vi "02 A_Setting a servo.vi"() -> ()   [LabVIEW 2019]
uses:
  _Subs/OpenDiagram/Open_XControl.xctl
  <vilib>/Instr/_visa.llb/VISA Configure Serial Port (Instr).vi
panel:
  in  "OpenDiag":refnum<vi>(xcontrol)
  out "position read":u8=100
  in  "Position":u8(slide)=98 scale=0.0..180.0
  in  "Arduino code":string="// include the Servo library\n#include <Servo.h>\n\nServo myServo;  // create a servo object\n\nvoid setup() {\n  myServo.attach(9); // attaches the servo on pin 9 to the servo object\n  Serial.begin(9600);\n\n}\n\nvoid loop() {   \n  int incomingByte;\n  if (Serial.available() > 0) {\n    int incomingByte = Serial.read();\n    myServo.write(incomingByte);\n    Serial.write(incomingByte);\n  }\n}"
  in  "stop":bool
  out "Connected":bool
  in  "Arduino Port":refnum<visa-resource-name>="ASRL26::INSTR"
  # "02 Arduino Setting  a Servo\nThis code takes will send a setting to your Arduino\n\nInstructions:\n1. Download the Arduino Code (SimpelServo) into your Arduino using the Arduino IDE\n2. Select the Arduino port \n3. Hit Run - and move the position slider"
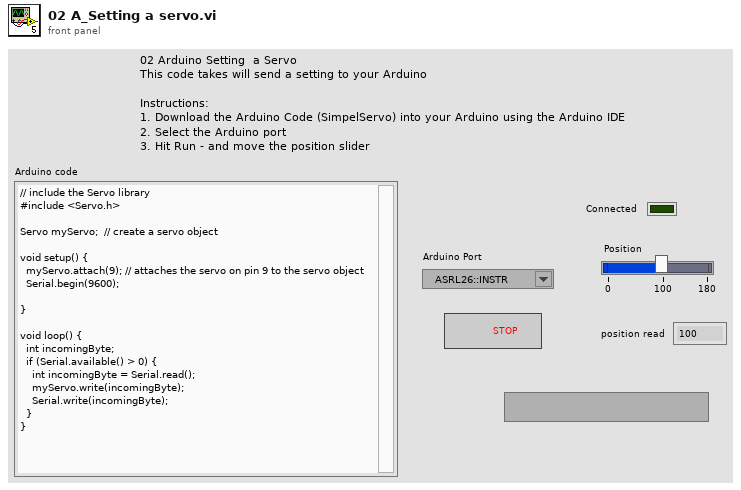
[diagram p1: front panel]
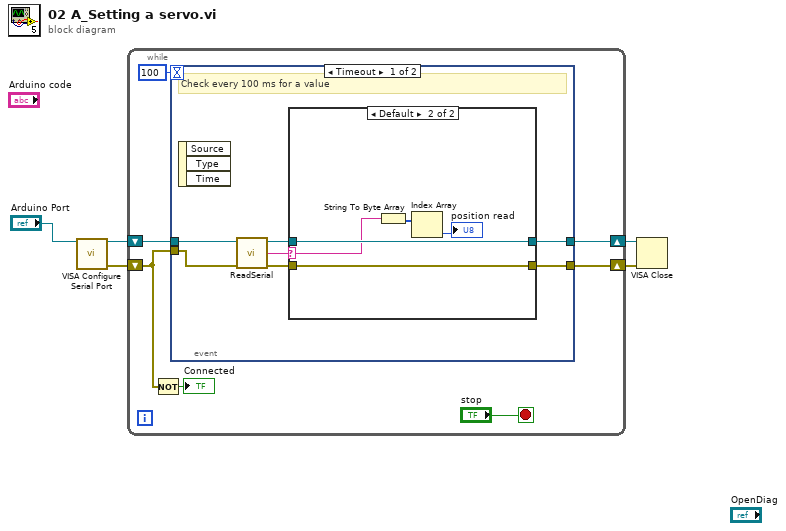
[diagram p0: block diagram]
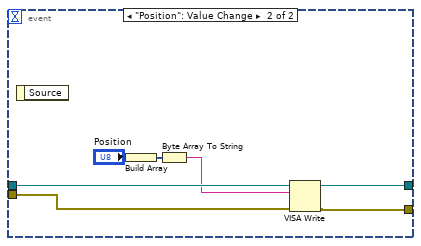
[diagram p3: hidden frame]
diagram:
  n1 = call-poly "VISA Configure Serial Port"("VISA resource name"="Arduino Port") -> ("VISA resource name out"=w4:refnum<visa-resource-name>, "error out"=w3:errorcluster)  [unwired: 13 in]
  n2 = while {
    shift-right: [w10] -> w1
    shift-left: w4 -> [w12]
    shift-right: [w11] -> w2
    shift-left: w3 -> [w8]
    stop <- "stop" stop-if-true
    n3 = Not(x=w8) -> (.not. x?=→"Connected":bool)
    n4 = event shown="[0] Timeout" {
      selector: _ -> [_ _]
      dyn-events: _ -> [_ _]
      timeout: 100 -> [_ _]
      tunnel: w12 -> [w17 w33]
      tunnel: [w19 w31] -> w11
      tunnel: [w18 w30] -> w10
      tunnel: w8 -> [w16 w32]
      event Timeout {
        # "Check every 100 ms for a value"
        n5 = event-data() -> ()  [unwired: 1 in, 3 out]
        n6 = call "ReadSerial.vi"("error in (no error)"=w16, "VISA Refnum in"=w17) -> ("error out"=w14:errorcluster, "String"=w13:string, "VISA Refnum out"=w15:refnum<visa-resource-name>)  [unwired: 7 in]
        n7 = case shown="Default" w13 {
          selector: w13 -> [_ w22]
          tunnel: [w20 w23] -> w19
          tunnel: [w21 w24] -> w18
          tunnel: w15 -> [w21 w24]
          tunnel: w14 -> [w20 w23]
          frame "" {
          }
          frame Default {
            n8 = String To Byte Array(string=w22) -> (unsigned byte array=w26:u8[])
            n9 = Index Array(array=w26) -> (element=→"position read":u8)  [unwired: 1 in]
          }
        }
      }
      event "Position": Value Change {
        n10 = event-data() -> ()  [unwired: 1 in, 1 out]
        n11 = Build Array("Position") -> (w28:u8[])
        n12 = Byte Array To String(unsigned byte array=w28) -> (string=w27:string)
        n13 = VISA Write(VISA resource name=w33, write buffer=w27, error in (no error)=w32) -> (VISA resource name out=w30:refnum<visa-resource-name>, error out=w31:errorcluster)  [unwired: 1 out]
      }
    }
  }
  n14 = VISA Close(VISA resource name=w1, error in (no error)=w2) -> ()  [unwired: 1 out]
